vi "Main_22A.vi"() -> ()   [LabVIEW 2024]
uses:
  Utility/Universal Utility/TypeDefs_Utility/Cluster_Row-Column.ctl
  9e3f57c0-2ef8-4495-8287-c6a42a5fb955.vi
  Utility/Universal Utility/TypeDefs_Utility/ENUM_4 Directions U-D-L-R.ctl
  Utility/Universal Utility/TypeDefs_Utility/ENUM_8 Directions U-D-L-R.ctl
panel:
  out "Secret Number Array":u64[](array[numeric])
  in  "Select Data":enum32{"Example", "Puzzle"}(tab)
  in  "Example":string="1\n10\n100\n2024"
  in  "Puzzle":string="8165752\n14569926\n3767076\n15353339\n2278086\n9212326\n11684913\n231995\n2939267\n13627562\n2230384\n8285292\n7154741\n1285944\n10343047\n13657793\n4654515\n4206420\n8850944\n6610095\n15413502\n16175073\n8854824\n7207123\n5868632\n11760123\n15172836\n2559018\n3890759\n6229173\n1236683\n9751316\n13463975\n6702739\n5888347\n4933103\n515922\n8949450\n16494878\n7532915\n11588505\n2130951\n1282099\n5405800\n7240657\n6907112\n16733850\n14934550\n5440328\n9388204\n15067401\n9916468\n15171410\n1793733\n3043612\n11049516\n12170977\n14260981\n9919481\n5861152\n7643802\n10656646\n13662054\n10162771\n10591940\n14303433\n11445420\n3767153\n970576\n6259366\n12730200\n8678271\n..."
  out "Answer":u32
  # "2000th"
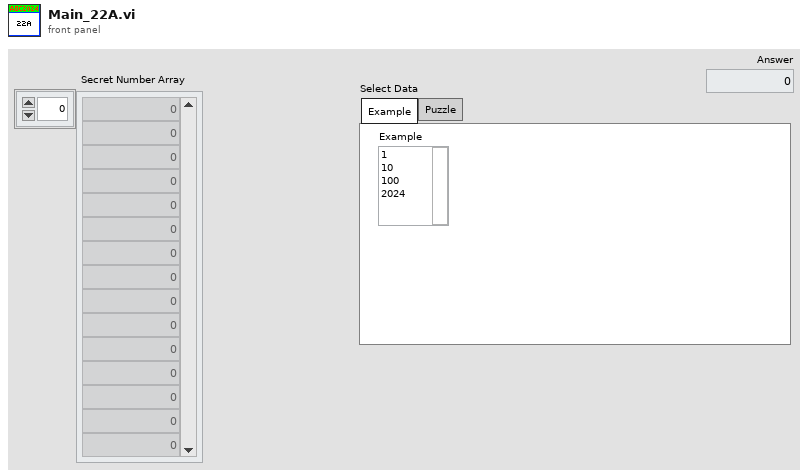
[diagram p1: front panel]
types:
  T1 = typedef "ENUM_8 Directions U-D-L-R.ctl" = enum16{"Up;-1,0", "Up-Right;-1,1", "Right;0,1", "Down-Right;1,1", "Down;1,0", "Down-Left;1,-1", "Left;0,-1", "Up-Left;-1,-1"}
  T2 = typedef "ENUM_4 Directions U-D-L-R.ctl" = enum16{"Up;-1,0", "Right;0,1", "Down;1,0", "Left;0,-1"}
  T3 = typedef "Cluster_Row-Column.ctl" = cluster{"R":i32, "C":i32}
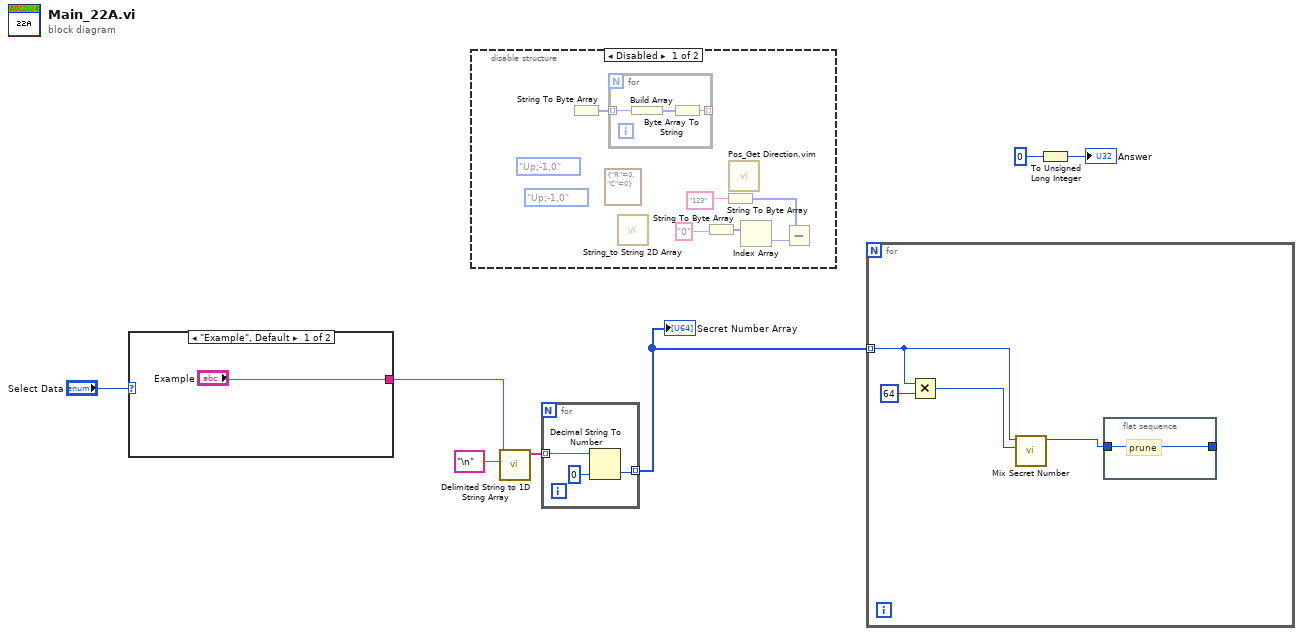
[diagram p0: block diagram]
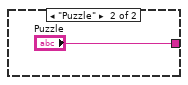
[diagram p2: hidden frame]
diagram:
  n1 = case shown="\"Example\", Default" "Select Data" {
    tunnel: ["Example" "Puzzle"] -> w2
    frame "Example", Default {
    }
    frame "Puzzle" {
    }
  }
  n2 = disable-structure shown="Disabled" {
    frame Disabled {
      (unwired) ENUM_8_Directions_U-D-L-R."Up;-1,0" ("Direction 8")
      (unwired) ENUM_4_Directions_U-D-L-R."Up;-1,0" ("Direction")
      (unwired) T3 {"R"=0, "C"=0} ("Position")
      n3 = String To Byte Array() -> (unsigned byte array=w10:u8[])  [unwired: 1 in]
      n4 = for {
        tunnel: w10 -> [w18] mode=indexing
        tunnel: [w16] -> _ mode=indexing
        n5 = Build Array(w18) -> (w17:u8[])
        n6 = Byte Array To String(unsigned byte array=w17) -> (string=w16:string)
      }
      n7 = call "String_to String 2D Array.vi"() -> ()  [unwired: 11 in, 1 out]
      n8 = String To Byte Array(string="0") -> (unsigned byte array=w13:u8[])
      n9 = String To Byte Array(string="123") -> (unsigned byte array=w11:u8[])
      n10 = call "Pos_Get Direction.vim"() -> ()  [unwired: 11 in, 1 out]
      n11 = Index Array(array=w13) -> (element=w12:u8)  [unwired: 1 in]
      n12 = Subtract(x=w11, y=w12) -> ()  [unwired: 1 out]
    }
    frame Enabled {
    }
  }
  n13 = call <vilib>:"Delimited String to 1D String Array.vi"("delimiter"="\n" ("delimiter (Tab)"), "delimited string"=w2) -> ("string array"=w6:string[])  [unwired: 9 in]
  n14 = for {
    tunnel: w6 -> [w21] mode=indexing
    tunnel: [w19] -> w1 mode=indexing
    n15 = Decimal String To Number(string=w21, default (0L)=u64 0 ("default (0 I32)")) -> (number=w19:u64)  [unwired: 1 in, 1 out]
  }
  "Secret Number Array" <- w1
  n16 = for {
    tunnel: w1 -> [w23] mode=indexing
    n17 = Multiply(x=w23, y=u64 64) -> (x*y=w24:u64)
    n18 = call "Mix Secret Number.vi"("Value"=w24, "Current Secret Number"=w23) -> ("New Secret Number"=w22:u64)  [unwired: 9 in]
    n19 = flat-sequence {
      tunnel: w22 -> [w26]
      tunnel: [w26] -> _
      frame #0 {
        # "prune"
      }
    }
  }
  n20 = To Unsigned Long Integer(number=u32 0) -> (unsigned 32bit integer=→"Answer":u32)
